vi "Module Not Running--error.vi"() -> (0 "error out":errorcluster)   [LabVIEW 2024, in "Cloneable Subpanel.lvlib"]
doc: "Outputs an error cluster containing a custom error code indicating the module is not running.\n_____\nBased on DQMH Dev Tools: Project Template 7.1.0.1499."
uses:
  Cloneable Subpanel.lvlib
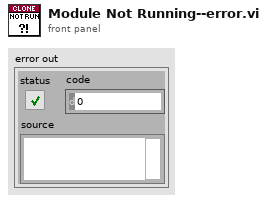
[diagram p1: front panel]
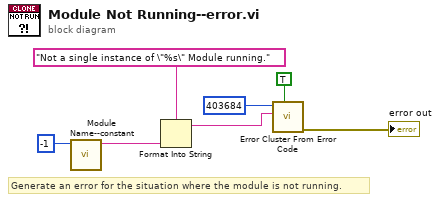
[diagram p0: block diagram]
diagram:
  # "Generate an error for the situation where the module is not running."
  n1 = call "Module Name--constant.vi"("Module ID"=-1) -> ("Module Name"=w2:string)  [unwired: 10 in]
  n2 = Format Into String(format string="Not a single instance of \"%s\" Module running.", w2) -> (resulting string=w6:string)  [unwired: 2 in, 1 out]
  n3 = call <vilib>:"Error Cluster From Error Code.vi"("show call chain? (False)"=TRUE, "error message (\"\")"=w6, "error code (0)"=403684) -> ("error out"=→"error out":errorcluster)  [unwired: 6 in]
